vi "App.vi"() -> ()   [LabVIEW 2022 SP3, in "Demo.lvlib"]
uses:
  Demo.lvlib
  Shared/Controls/Global.ctl
  Shared/Shared.lvlib
  <vilib>/Utility/LVLibp/NI_PackedLibraryUtility.lvlib
  Test1/Test1.lvlib
panel:
  out "call chain":string[](array[string])
  out "error out 2":errorcluster
  out "Dependency Paths":path[](array[path])
  out "Dependency Names":string[](array[string])
  out "x+y":dbl
  in  "x":dbl
  in  "y":dbl
  out "qualified names":string[](array[string])
  out "paths":path[](array[path])
  out "error out":errorcluster
  out "packed library path":path
  out "Is In Packed Library":bool
  out "Application:All VIs In Memory":string[](array[string])
  out "Application:All Libraries in Application Instance":string[](array[string])
  out "Ticks":u32
  out "Self":T1
  in  "_Exit":bool
  out "Instances":T1[](array[typedef])
  in  "ID":i32
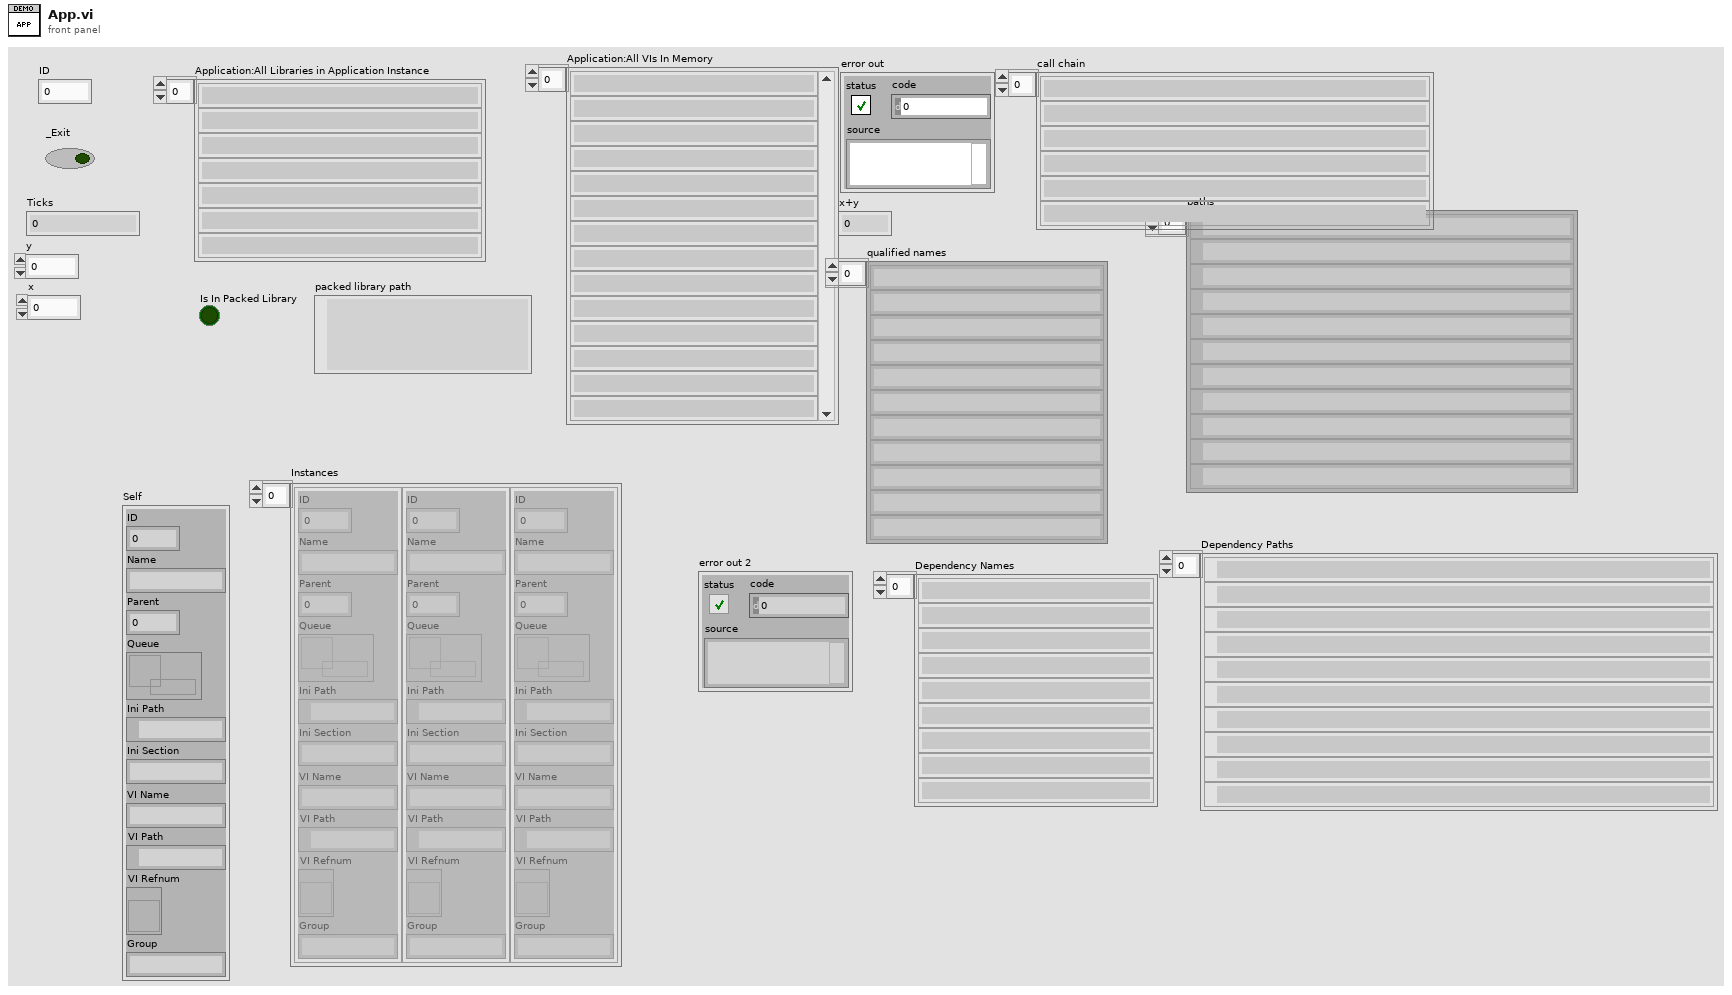
[diagram p1: front panel]
types:
  T1 = typedef "Shared.lvlib/Global.ctl" = cluster{"ID":i32, "Name":string, "Parent":i32, "Queue":refnum<queue>, "Ini Path":path, "Ini Section":string, "VI Name":string, "VI Path":path, "VI Refnum":refnum<vi>, "Group":string}
  T2 = enum8{"Include the clone VI", "Include the original reentrant VI instead of the clone VI", "Include both the original reentrant VI and the clone VI"}
  T3 = enum8{"No dynamic dispatch VIs", "Include nearest implementation", "Include all overrides"}
  T4 = enum8{"Only include commented out diagrams if diagram already loaded", "Never include commented out diagrams", "Always include commented out diagrams"}
  T5 = typedef "Shared.lvlib/Instance.ctl" = cluster{"ID":i32, "Queue":refnum<queue>, "Global":refnum<k1>}
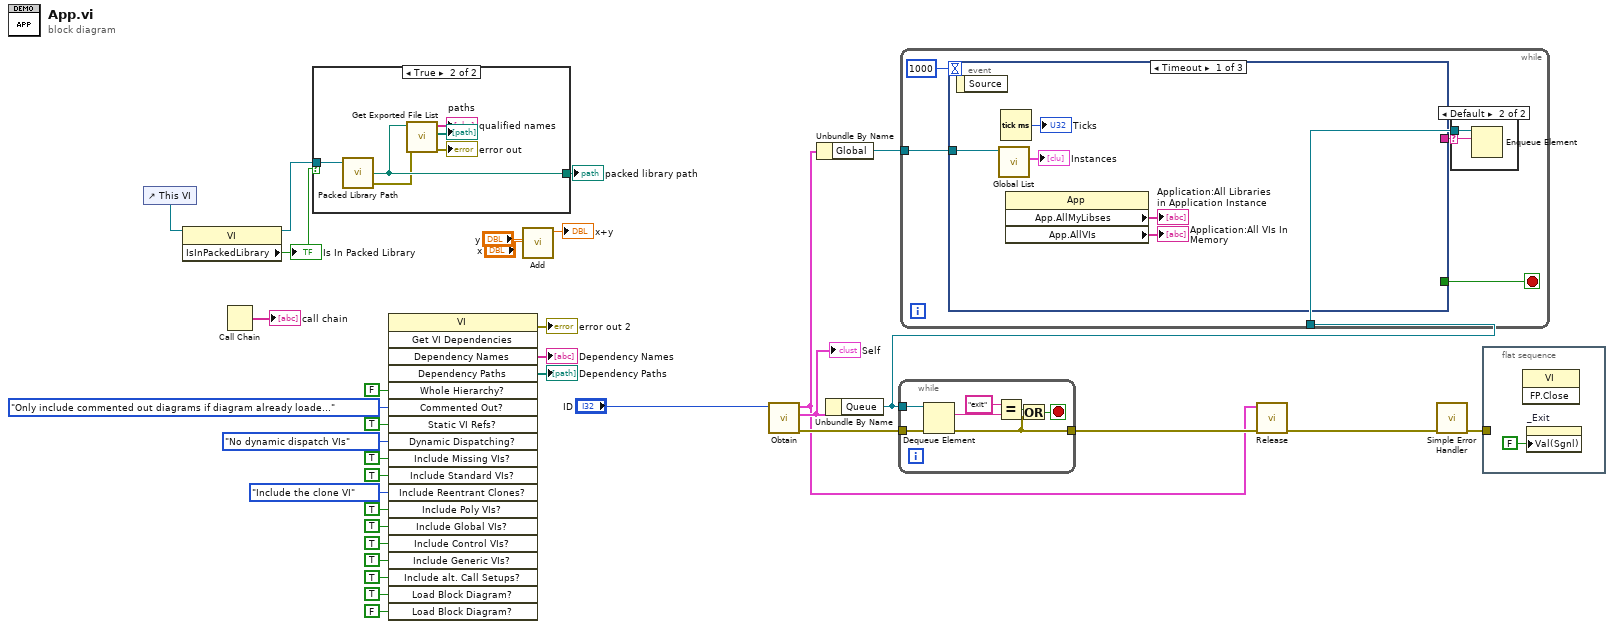
[diagram p0: block diagram]
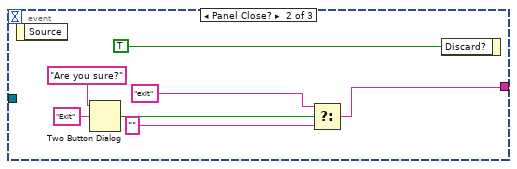
[diagram p4: hidden frame]
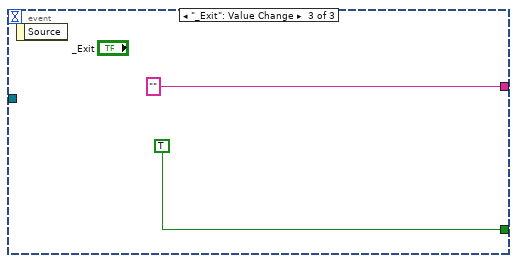
[diagram p5: hidden frame]
diagram:
  n1 = control-ref of="This VI"() -> (w25:refnum<vi>)
  n2 = property class="VI"(reference=w25) -> (reference out=w19:refnum<vi>, "IsInPackedLibrary"=w24:bool)  [unwired: 1 in, 1 out]
  "Is In Packed Library" <- w24
  n3 = Call Chain() -> (call chain=→"call chain":string[])
  n4 = case shown="True" w24 {
    tunnel: w19 -> [_ w40]
    tunnel: [_ w39] -> w23
    frame False {
    }
    frame True {
      n5 = call <vilib>:"Packed Library Path.vi"("vi reference"=w40) -> ("error out"=w38:errorcluster, "packed library path"=w39:path)  [unwired: 2 in, 1 out]
      n6 = call <vilib>:"Get Exported File List.vi"("error in (no error)"=w38, "packed library path"=w39) -> ("error out"=→"error out":errorcluster, "paths"=→"paths":path[], "qualified names"=→"qualified names":string[])  [unwired: 7 in]
    }
  }
  "packed library path" <- w23
  n7 = invoke class="VI" method="Get VI Dependencies"("Whole Hierarchy?"=FALSE, "Commented Out?"=T4."Only include commented out diagrams if diagram already loaded" ("Commented Out Diagrams?"), "Static VI Refs?"=TRUE, "Dynamic Dispatching?"=T3."No dynamic dispatch VIs", "Include Missing VIs?"=TRUE ("Include Missing Items?"), "Include Standard VIs?"=TRUE, "Include Reentrant Clones?"=T2."Include the clone VI", "Include Poly VIs?"=TRUE, "Include Global VIs?"=TRUE, "Include Control VIs?"=TRUE, "Include Generic VIs?"=TRUE, "Include alt. Call Setups?"=TRUE ("Include Alternate Call Setups?"), "Load Block Diagram?"=TRUE ("Keep Express and Malleable VIs?"), "Load Block Diagram?"=FALSE) -> (error out=→"error out 2":errorcluster, "Dependency Names"=→"Dependency Names":string[], "Dependency Paths"=→"Dependency Paths":path[])  [unwired: 5 in, 16 out]
  n8 = call "Add.vi"("y"="y", "x"="x") -> ("x+y"=→"x+y":dbl)  [unwired: 9 in]
  n9 = call "Obtain.vi"("ID in"="ID") -> ("error out"=w32:errorcluster, "Self"=w31:T1, "Instance"=w29:T5)  [unwired: 8 in]
  "Self" <- w31
  n10 = Unbundle By Name(w29) -> ("Global"=w28:refnum<k1>)
  n11 = Unbundle By Name(w31) -> ("Queue"=w30:refnum<queue>)
  n12 = while {
    tunnel: w30 -> [w47]
    tunnel: w32 -> [w46]
    tunnel: [w41] -> w33
    stop <- w42 stop-if-true
    n13 = Dequeue Element(queue=w47, error in (no error)=w46) -> (element=w45:string, error out=w41:errorcluster)  [unwired: 1 in, 2 out]
    n14 = Equal?(x="exit" ("y"), y=w45) -> (x = y?=w43:bool)
    n15 = Or(x=w43, y=w41) -> (x .or. y?=w42:bool)
  }
  n16 = while {
    tunnel: w30 -> [w52]
    tunnel: w28 -> [w48]
    stop <- w51 stop-if-true
    n17 = event shown="[0] Timeout" {
      selector: _ -> [_ _ _]
      dyn-events: _ -> [_ _ _]
      timeout: 1000 -> [_ _ _]
      tunnel: [_ _ TRUE] -> w51
      tunnel: [_ w60 "" ("element")] -> w50
      tunnel: w48 -> [w59 _ _]
      event Timeout {
        n18 = event-data() -> ()  [unwired: 1 in, 1 out]
        n19 = call "Global List.vi"("Global in"=w59) -> ("Instances"=→"Instances":T1[])  [unwired: 8 in, 2 out]
        n20 = Tick Count (ms)() -> (millisecond timer value=→"Ticks":u32)
        n21 = property class="App"() -> ("App.AllMyLibses"=→"Application:All Libraries in Application Instance":string[], "App.AllVIs"=→"Application:All VIs In Memory":string[])  [unwired: 2 in, 2 out]
      }
      event Panel Close? {
        n22 = event-data() -> ()  [unwired: 1 in, 1 out]
        n23 = Two Button Dialog(message="Are you sure?", 2:"Exit" ("T button name (\"OK\")")) -> (T button?=w63:bool)  [unwired: 1 in]
        n24 = Select(t="exit", s=w63, f="") -> (s? t:f=w60:string)
        n25 = event-data("Discard?"=TRUE) -> ()  [unwired: 1 in, 1 out]
      }
      event "_Exit": Value Change {
        n26 = event-data() -> ()  [unwired: 1 in, 1 out]
      }
    }
    n27 = case shown="Default" w50 {
      selector: w50 -> [_ w53]
      tunnel: w52 -> [_ w54]
      frame "" {
      }
      frame Default {
        n28 = Enqueue Element(queue=w54, element=w53) -> ()  [unwired: 2 in, 3 out]
      }
    }
  }
  n29 = call "Release.vi"("error in (no error)"=w33, "Instance"=w29) -> ("error out"=w27:errorcluster)  [unwired: 8 in, 1 out]
  n30 = call <vilib>:"Simple Error Handler.vi"("error in (no error)"=w27) -> ("error out"=w26:errorcluster)  [unwired: 4 in, 4 out]
  n31 = flat-sequence {
    tunnel: w26 -> [_]
    frame #0 {
      n32 = invoke class="VI" method="FP.Close"() -> ()  [unwired: 3 in, 3 out]
      n33 = property on="_Exit" class="Bool (strict)"("Val(Sgnl)"=FALSE ("Value (Signaling)")) -> ()  [unwired: 2 in, 2 out]
    }
  }
